vi "Create MC Cycle Engine Actual Message Data .vi"(2 "Cycle #":u8, 7 "MC Cycle Engine State":T1, 11 "Error In":errorcluster) -> (4 "MC Cycle Engine Request Message Data":string, 15 "Error Out":errorcluster)   [LabVIEW 2016, in "TLMB.lvlib"]
doc: "This vi should be used to generate the Message Data for changing the MC Cycle Engine States."
uses:
  Projects/TLMB.lvlib
  type defs/MC_Cycle_Engine_Actual_State.ctl
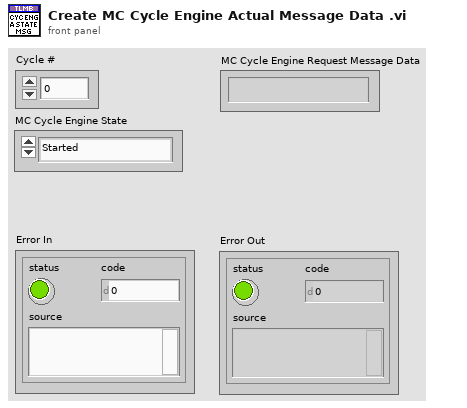
[diagram p1: front panel]
types:
  T1 = typedef "TLMB.lvlib/MC_Cycle_Engine_Actual_State.ctl" = enum16{"Started", "Stopped", "Paused", "Resumed", "Selected", "Completed"}
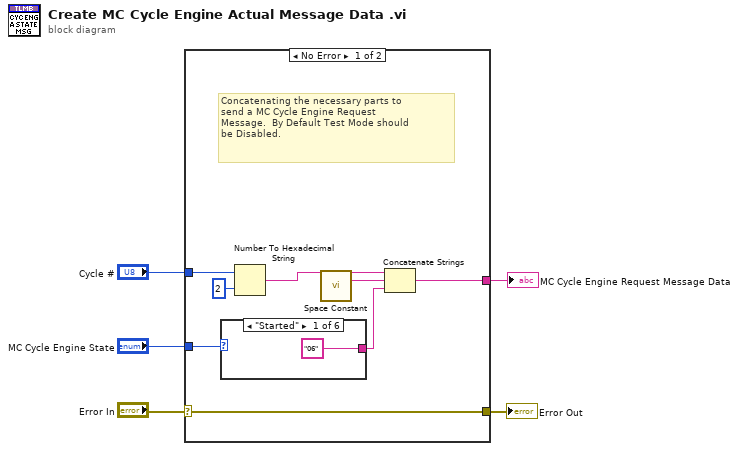
[diagram p0: block diagram]
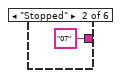
[diagram p2: hidden frame]
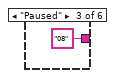
[diagram p3: hidden frame]
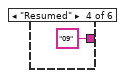
[diagram p4: hidden frame]
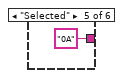
[diagram p5: hidden frame]
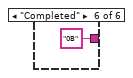
[diagram p6: hidden frame]
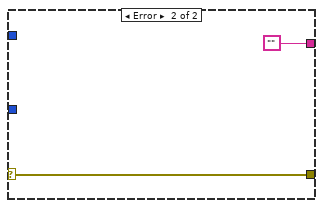
[diagram p7: hidden frame]
diagram:
  n1 = case shown="No Error" "Error In" {
    selector: "Error In" -> [w12 w20]
    tunnel: "MC Cycle Engine State" -> [w13 _]
    tunnel: [w12 w20] -> w3
    tunnel: "Cycle #" -> [w11 _]
    tunnel: [w8 ""] -> w1
    frame No Error {
      # "Concatenating the necessary parts to\nsend a MC Cycle Engine Request \nMessage.  By Default Test Mode should\nbe Disabled."
      n2 = case shown="\"Started\"" w13 {
        tunnel: ["06" ("Message") "07" ("Message") "08" ("Message") "09" ("Message") "0A" ("Message") "0B" ("Message")] -> w9
        frame "Started" {
        }
        frame "Stopped" {
        }
        frame "Paused" {
        }
        frame "Resumed" {
        }
        frame "Selected" {
        }
        frame "Completed" {
        }
      }
      n3 = Number To Hexadecimal String(1:i16 2 ("width (-)"), 2:w11) -> (0:w6:string)
      n4 = call <vilib>:"Space Constant.vi"() -> ("String"=w7:string)
      n5 = Concatenate Strings(w6, w7, w9) -> (w8:string)
    }
    frame Error {
    }
  }
  "Error Out" <- w3
  "MC Cycle Engine Request Message Data" <- w1
